vi "TicMove-temp.vi"() -> ()   [LabVIEW 2018]
panel:
  in  "Address":u16=16384 caption="Address [16384=Unadressed]" max=16384
  out "Numeric":i32
  in  "Target (Pulses)":i32
  in  "VISA resource name":refnum<visa-resource-name>
  out "Position(pulses)":i32
  in  "moveTimeout(s)":dbl=60.0
  in  "readInterval(ms)":u32=100
  out "Time(s)":dbl
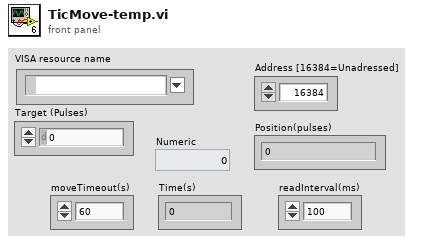
[diagram p1: front panel]
types:
  T1 = enum16{"GetStatus", "GetPosition", "SetTarget", "Enable", "Disable", "SetCurrent", "GetVelocity", "GetUptime", "GetVsupply", "Reset", "Go"}
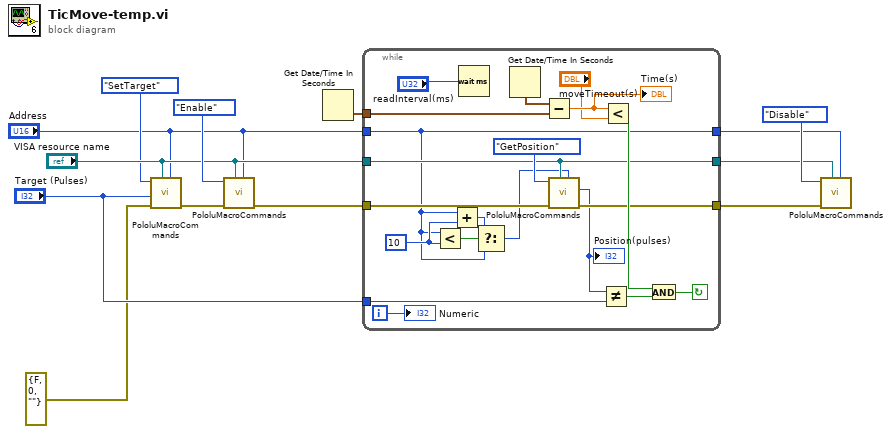
[diagram p0: block diagram]
diagram:
  n1 = call "PololuMacroCommands.vi"("Address"="Address", "VISA resource name"="VISA resource name", "Error In"=errorcluster {"status"=FALSE, "code"=0, "source"=""}, "Argument"="Target (Pulses)", "Procedure"=T1."SetTarget" ("Enum")) -> ("Error Out"=w8:errorcluster)  [unwired: 4 in, 2 out]
  n2 = call "PololuMacroCommands.vi"("Address"="Address", "VISA resource name"="VISA resource name", "Error In"=w8, "Procedure"=T1."Enable" ("Enum")) -> ("Error Out"=w9:errorcluster)  [unwired: 5 in, 2 out]
  n3 = Get Date/Time In Seconds() -> (seconds since 1Jan1904=w13:timestamp)
  n4 = while {
    tunnel: w9 -> [w32]
    tunnel: "VISA resource name" -> [w21]
    tunnel: "Target (Pulses)" -> [w30]
    tunnel: w13 -> [w28]
    tunnel: [w23] -> w12
    tunnel: [w21] -> w10
    tunnel: "Address" -> [w15]
    tunnel: [w15] -> w2
    i -> [w19]
    stop <- w25 continue-if-true
    w18 = u16 10 ("y")
    n5 = Less?(x=w15, y=w18) -> (x < y?=w17:bool)
    n6 = Add(x=w15, y=w18) -> (x+y=w16:u16)
    n7 = Wait (ms)(milliseconds to wait="readInterval(ms)") -> ()  [unwired: 1 out]
    n8 = Select(t=w16, s=w17, f=w15) -> (s? t:f=w14:u16)
    n9 = Get Date/Time In Seconds() -> (seconds since 1Jan1904=w29:timestamp)
    n10 = Subtract(x=w29, y=w28) -> (x-y=w27:dbl)
    "Time(s)" <- w27
    n11 = call "PololuMacroCommands.vi"("Address"=w14, "VISA resource name"=w21, "Error In"=w32, "Procedure"=T1."GetPosition" ("Enum")) -> ("Error Out"=w23:errorcluster, "32-bitReadValue"=w20:i32)  [unwired: 5 in, 1 out]
    "Position(pulses)" <- w20
    n12 = Not Equal?(x=w20, y=w30) -> (x != y?=w33:bool)
    n13 = Less?(x=w27, y="moveTimeout(s)") -> (x < y?=w24:bool)
    n14 = And(x=w24, y=w33) -> (x .and. y?=w25:bool)
    "Numeric" <- w19
  }
  n15 = call "PololuMacroCommands.vi"("Address"=w2, "VISA resource name"=w10, "Error In"=w12, "Procedure"=T1."Disable" ("Enum")) -> ()  [unwired: 5 in, 3 out]
